vi "Join U16.vi"(7 "LSB Length":u8=4, 10 "LSB":u16 format="%x", 11 "MSB":u16 format="%x") -> (3 "U16":u16 format="%x")   [LabVIEW 2021, in "DataTypes_CIF_U.lvlib"]
doc: "This will split a byte into two numbers each using a subset of the bits. The MSB for Ethernet is the portion of the byte that contains bit 0."
uses:
  DataTypes_CIF_U.lvlib
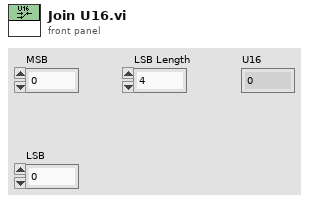
[diagram p1: front panel]
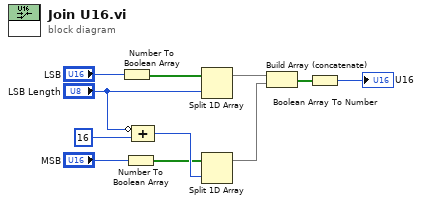
[diagram p0: block diagram]
diagram:
  n1 = Number To Boolean Array(number="LSB") -> (Boolean array=w10:bool[])
  n2 = Number To Boolean Array(number="MSB") -> (Boolean array=w3:bool[])
  n3 = Compound Arithmetic op=ADD(invert "LSB Length", u8 16 ("value")) -> (w9:u8)
  n4 = Split 1D Array(array=w10, index="LSB Length") -> (first subarray=w8:bool[])  [unwired: 1 out]
  n5 = Split 1D Array(array=w3, index=w9) -> (first subarray=w2:bool[])  [unwired: 1 out]
  n6 = Build Array (concatenate)(w8, w2) -> (w7:bool[])
  n7 = Boolean Array To Number(Boolean array=w7) -> (number=→"U16":u16)
